vi "start.vi"(8 "error in (no error)":errorcluster, 11 "manager_daemon in":refnum<class "manager_daemon.lvclass">) -> (0 "error out":errorcluster, 3 "manager_daemon out":refnum<class "manager_daemon.lvclass">)   [LabVIEW 2024, in "manager_daemon.lvclass"]
uses:
  manager_daemon.lvclass
  private/daemon.vi
  manager_daemon.lvclass/manager_daemon.ctl
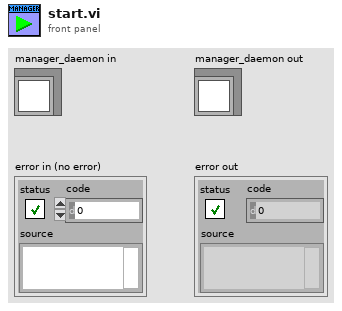
[diagram p1: front panel]
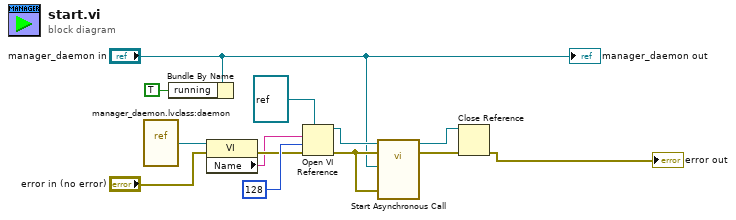
[diagram p0: block diagram]
diagram:
  n1 = vi-ref "manager_daemon.lvclass:daemon.vi"() -> (w12:refnum<vi>)
  n2 = Bundle By Name(cluster="manager_daemon in", "running"=TRUE) -> ()  [unwired: 1 out]
  n3 = property class="VI"(reference=w12, error in="error in (no error)") -> (error out=w11:errorcluster, "Name"=w10:string)  [unwired: 1 out]
  n4 = Open VI Reference(type specifier VI Refnum (for type only)=refnum<vi> refnum, vi path=w10, options=128, error in (no error)=w11) -> (vi reference=w8:refnum<vi>, error out=w5:errorcluster)  [unwired: 2 in]
  n5 = call-by-ref "Start Asynchronous Call"(reference=w8, error in=w5, 8:"error in (no error)"=w5, "manager_daemon.lvclass"="manager_daemon in") -> (reference out=w7:refnum<vi>, error out=w6:errorcluster)  [unwired: 10 in]
  n6 = Close Reference(reference=w7, error in (no error)=w6) -> (error out=→"error out":errorcluster)
  "manager_daemon out" <- "manager_daemon in"
